vi "Sim Engine.vi"() -> ()   [LabVIEW 2013]
uses:
  <vilib>/NI/Module Execution Interface/Engine Runtime/Execution States.ctl
  <vilib>/NI/Module Execution Interface/Engine Runtime/Engine Runtime Interface.lvclass
  <vilib>/NI/Tag Bus Data Framework/Framework Configuration Classes/target runtime/PL_Target Runtime.lvclass
  <vilib>/NI/Configuration Framework/tree serializer/NISE_CEF_TreeSerializer.lvlib
  <vilib>/NI/Tag Bus Data Framework/Framework Configuration Classes/flattened data interface/PL_Serialization Interface.lvlib
  <vilib>/NI/TBM Engines/Standard Engine/Runtime/Standard Engine Runtime.lvclass
panel:
  in  "file path":path=path "C:/TBD/Sample Applications/RT Temperature Controller/SimulatedSystem.pcfg"
  out "final error":errorcluster
  in  "stop":bool
  out "runtime error":errorcluster
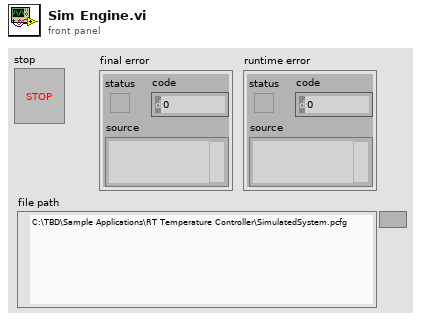
[diagram p1: front panel]
types:
  T1 = typedef "NISE_CEF_TreeSerializer.lvlib/base file format.ctl" = cluster{"version":string, "data":string}
  T2 = typedef "NISE_CEF_TreeSerializer.lvlib/flat hierarchy.ctl" = cluster{"hierarchy structure":T3, "instance data":T5[]}
  T3 = typedef "NISE_CEF_TreeSerializer.lvlib/full hierarchy.ctl" = cluster{"root":string, "hierarchy":T4[]}
  T4 = typedef "NISE_CEF_TreeSerializer.lvlib/hierarchy element.ctl" = cluster{"current node":string, "children":string[]}
  T5 = typedef "NISE_CEF_TreeSerializer.lvlib/instance data.ctl" = cluster{"ID":string, "Alias":string, "class":string, "version":string, "data":string}
  T6 = typedef "PLConfigurationSerializer.lvlib/targets cluster.ctl" = cluster{"Target Configuration":refnum<class "PL_Target Configuration.lvclass">, "engines":T7[]}
  T7 = typedef "PLConfigurationSerializer.lvlib/engines cluster.ctl" = cluster{"engine configuration":refnum<class "engine configuration.lvclass">, "modules":refnum<class "TBM module configuration.lvclass">[]}
  T8 = typedef "Engine Runtime Interface.lvclass/Execution States.ctl" = enum16{"Initializing", "Paused (Initialized)", "Running", "Set Safe Outputs", "Uninitializing", "Stopped (Uninitialized)", "Error (Uninitialized)", "Safe State (Uninitialized)", "Closed"}
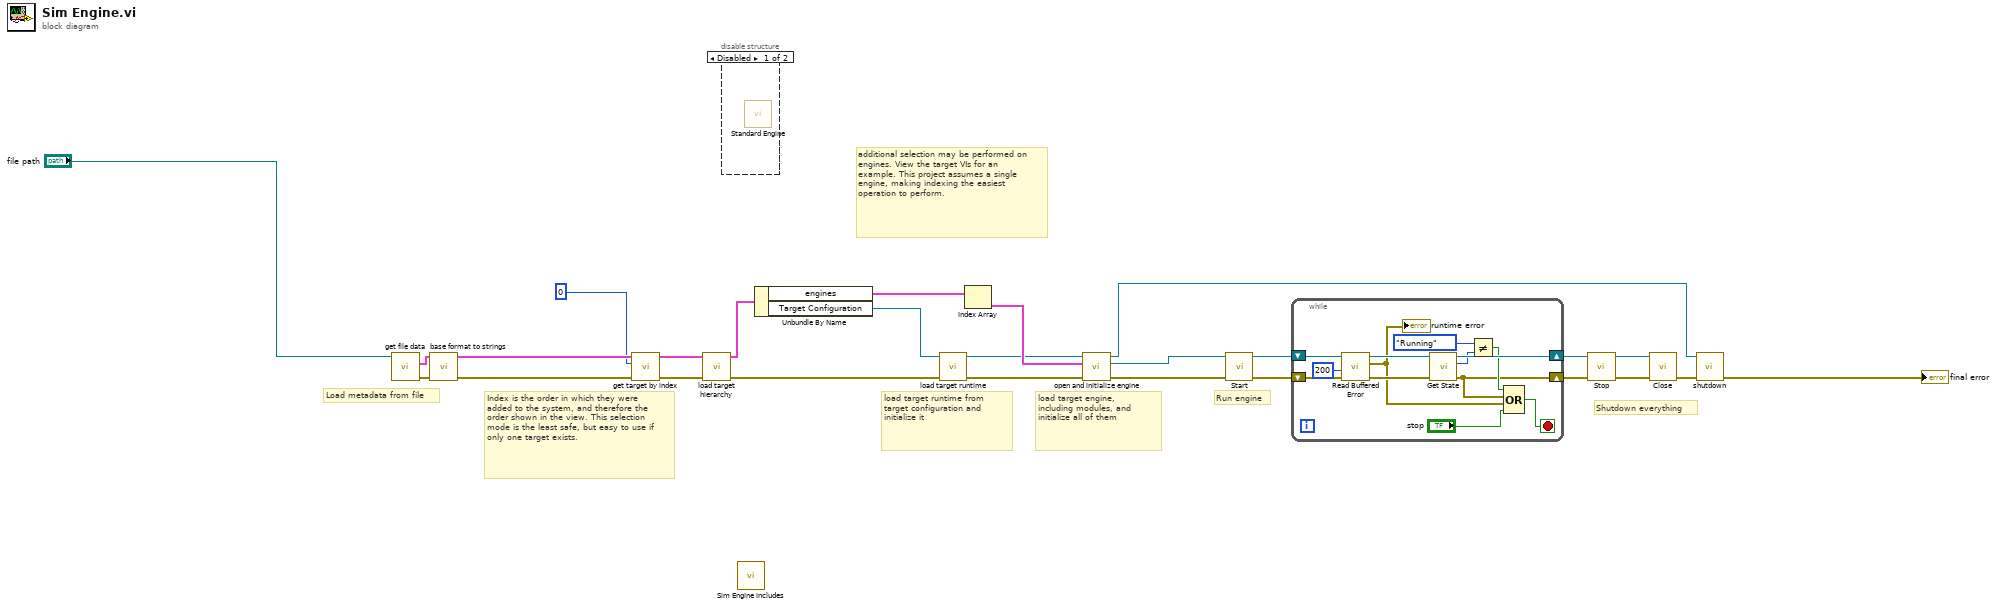
[diagram p0: block diagram]
diagram:
  # "Index is the order in which they were added to the system, and therefore the order shown in the view. This selection mode is the least safe, but easy to use if only one target exists."
  # "additional selection may be performed on engines. View the target VIs for an example. This project assumes a single engine, making indexing the easiest operation to perform."
  # "Shutdown everything"
  # "Run engine"
  # "load target engine, including modules, and initialize all of them"
  # "load target runtime from target configuration and initialize it"
  # "Load metadata from file"
  n1 = call <vilib>:"get file data.vi"("Path"="file path") -> ("error out"=w10:errorcluster, "format"=w9:T1)  [unwired: 9 in]
  n2 = call <vilib>:"base format to strings.vi"("error in"=w10, "format"=w9) -> ("error out"=w7:errorcluster, "data"=w6:T2)  [unwired: 8 in]
  n3 = call <vilib>:"get target by index.vi"("error in"=w7, "index"=0 ("target"), "system hierarchy"=w6) -> ("error out"=w4:errorcluster, "target hierarchy"=w5:T2)  [unwired: 7 in]
  n4 = call <vilib>:"load target hierarchy.vi"("error in"=w4, "target hierarchy"=w5) -> ("error out"=w3:errorcluster, "targets cluster out"=w2:T6)  [unwired: 8 in]
  n5 = disable-structure shown="Disabled" {
    frame Disabled {
      n6 = call <vilib>:"Standard Engine.vi"() -> ()  [unwired: 11 in, 1 out]
    }
    frame Enabled {
    }
  }
  n7 = call "Sim Engine Includes.vi"() -> ()  [unwired: 12 in]
  n8 = Unbundle By Name(w2) -> ("engines"=w20:T7[], "Target Configuration"=w14:refnum<class "PL_Target Configuration.lvclass">)
  n9 = call <vilib>:"load target runtime.vi"("error in"=w3, "target configuration"=w14) -> ("error out"=w13:errorcluster, "target runtime"=w12:refnum<class "PL_Target Runtime.lvclass">)  [unwired: 8 in]
  n10 = Index Array(array=w20) -> (element=w15:T7)  [unwired: 1 in]
  n11 = call <vilib>:"open and initialize engine.vi"("error in"=w13, "engine configuration in"=w15, "Target Runtime in"=w12) -> ("error out"=w19:errorcluster, "Engine Runtime Interface out"=w18:refnum<class "Engine Runtime Interface.lvclass">, "Target Runtime out"=w16:refnum<class "PL_Target Runtime.lvclass">)  [unwired: 6 in]
  n12 = call-dynamic "Start.vi"("error in"=w19, "Engine Runtime Interface in"=w18) -> ("error out"=w21:errorcluster, "Engine Runtime Interface out"=w24:refnum<class "Engine Runtime Interface.lvclass">)  [unwired: 8 in]
  n13 = while {
    shift-right: [w35] -> w23
    shift-left: w24 -> [w39]
    shift-right: [w28] -> w22
    shift-left: w21 -> [w38]
    stop <- w33 stop-if-true
    n14 = call-dynamic "Read Buffered Error.vi"("error in"=w38, "timeout in ms (0)"=200, "Engine Runtime Interface in"=w39) -> ("error out"=w36:errorcluster, "Engine Error"=w32:errorcluster, "Engine Runtime Interface out"=w37:refnum<class "Engine Runtime Interface.lvclass">)  [unwired: 6 in]
    "runtime error" <- w32
    n15 = call-dynamic "Get State.vi"("error in"=w36, "Engine Runtime Interface in"=w37) -> ("error out"=w28:errorcluster, "Engine State"=w31:T8, "Engine Runtime Interface out"=w35:refnum<class "Engine Runtime Interface.lvclass">)  [unwired: 7 in]
    n16 = Not Equal?(x=Execution_States."Running" ("Engine State"), y=w31) -> (x != y?=w29:bool)
    n17 = Compound Arithmetic op=OR(w29, w28, w32, "stop") -> (w33:bool)
  }
  n18 = call-dynamic "Stop.vi"("error in"=w22, "Engine Runtime Interface in"=w23) -> ("error out"=w25:errorcluster, "Engine Runtime Interface out"=w26:refnum<class "Engine Runtime Interface.lvclass">)  [unwired: 8 in]
  n19 = call-dynamic "Close.vi"("error in"=w25, "Engine Runtime Interface in"=w26) -> ("error out"=w17:errorcluster)  [unwired: 9 in]
  n20 = call-dynamic "shutdown.vi"("error in"=w17, "Target Runtime in"=w16) -> ("error out"=→"final error":errorcluster)  [unwired: 9 in]
